vi "Write Measurement Type.vi"(8 "error in":errorcluster, 10 "measurement type":T1, 11 "PWM input channel in":refnum<class "PWM Input Channel.lvclass">) -> (0 "error out":errorcluster, 3 "PWM input channel out":refnum<class "PWM Input Channel.lvclass">)   [LabVIEW 2020, in "Scan Engine Scripting.lvlib" / "PWM Input Channel.lvclass"]
uses:
  PWM Input Channel.lvclass
  Measurement Type.ctl
  PWM Input Channel.lvclass/PWM Input Channel.ctl
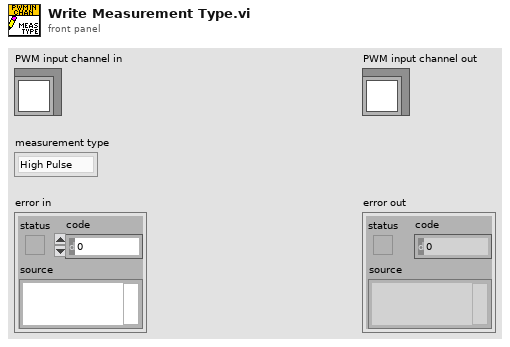
[diagram p1: front panel]
types:
  T1 = typedef "Scan Engine Scripting.lvlib/PWM Input Channel.lvclass/Measurement Type.ctl" = enum16{"High Pulse", "Low Pulse", "Most Recent"}
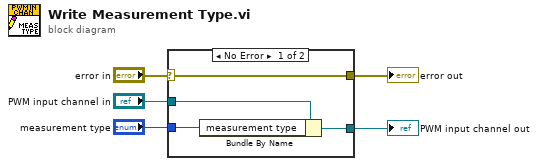
[diagram p0: block diagram]
diagram:
  n1 = case shown="No Error" "error in" {
    selector: "error in" -> [w9 w10]
    tunnel: [w9 w10] -> w4
    tunnel: [w7 w11] -> w2
    tunnel: "PWM input channel in" -> [w8 w11]
    tunnel: "measurement type" -> [w6 _]
    frame No Error {
      n2 = Bundle By Name(cluster=w8, "measurement type"=w6) -> (w7:refnum<class "PWM Input Channel.lvclass">)
    }
    frame Error {
    }
  }
  "error out" <- w4
  "PWM input channel out" <- w2
